vi "PathDrawerMain.vi"() -> ()   [LabVIEW 2017]
uses:
  Shared/PathFileData.ctl
  Shared/RobotNeededPathData.ctl
panel:
  in  "Tab Control":enum32{"Path", "Load/Save"}(tab)
  in  "Points":cluster{dbl, dbl}[](array[cluster])=[{46.0, 206.0}, {72.0, 199.0}, {97.0, 267.0}, {149.0, 262.0}]
  in  "Roundedness":dbl(slide)=0.7875252525252525 scale=0.6..0.995
  in  "RobotLength":dbl=40.0
  in  "RobotWidth":dbl=30.0
  in  "CenterOfRotYOffset":dbl=20.0
  in  "PointSpacing":dbl=12.0 min=1.0 format="%#_13g"
  in  "Starting Position Preset":enum16{"1", "2", "3", "4", "No Preset"}(ring)=enum."3"
  in  "Flip Path":bool
  in  "MaxVel":dbl=100.0 format="%#_13g"
  in  "MaxAccel":dbl=100.0 format="%#_13g"
  in  "LocalTempPaths":i32(listbox)
  out "standard output":string
  in  "ExportToLocal":bool
  in  "LoadFromLocal":bool
  in  "ExportToRobot":bool
  in  "LoadAllFromRobot":bool
  in  "LocalPaths":i32(listbox)
  out "standard error":string
  in  "LocalFileNames":string[](array[string])
  in  "Stop":bool
  out "Path Drawer":T1(plugin-control)
  # "MORE INSTRUCTIONS"
  # "Use a preset if your path starts\nat one of the presets. \n\n(Click it multiple times please)"
  # "Includes bumpers"
  # "Relative to outside face of\nback bumber of robot"
  # "INSTRUCTIONS"
  # "The red line is the path that the robot recieves. Everything else is to help create that path\n\nUse the multi-line tool to draw a path. Double click to stop drawing.\nHover over a node and press backspace to remove it.\nPress I to insert a new node (at the end of the path only, for now)\n\nUse the contols to input robot width, height, and center of rotation offset,\nHow far apart the points in the \"real world units\" path are,\nWhether the robot travels on the left or right of your green lines, and\nthe roundedness of the path. (Note: point spacing affects roundedness)\n\nYou can manually edit the green node's location in the path with the Points array,\nor drag the nodes on the image\n\nPress Export To File and enter the file name (no extension) to save the path to a file in the\nThisVIsDirectory\\Paths\\ folder\n\nIf you acidentally clear your path press Z quickly to get it back"
  # "Responses of CMDs run"
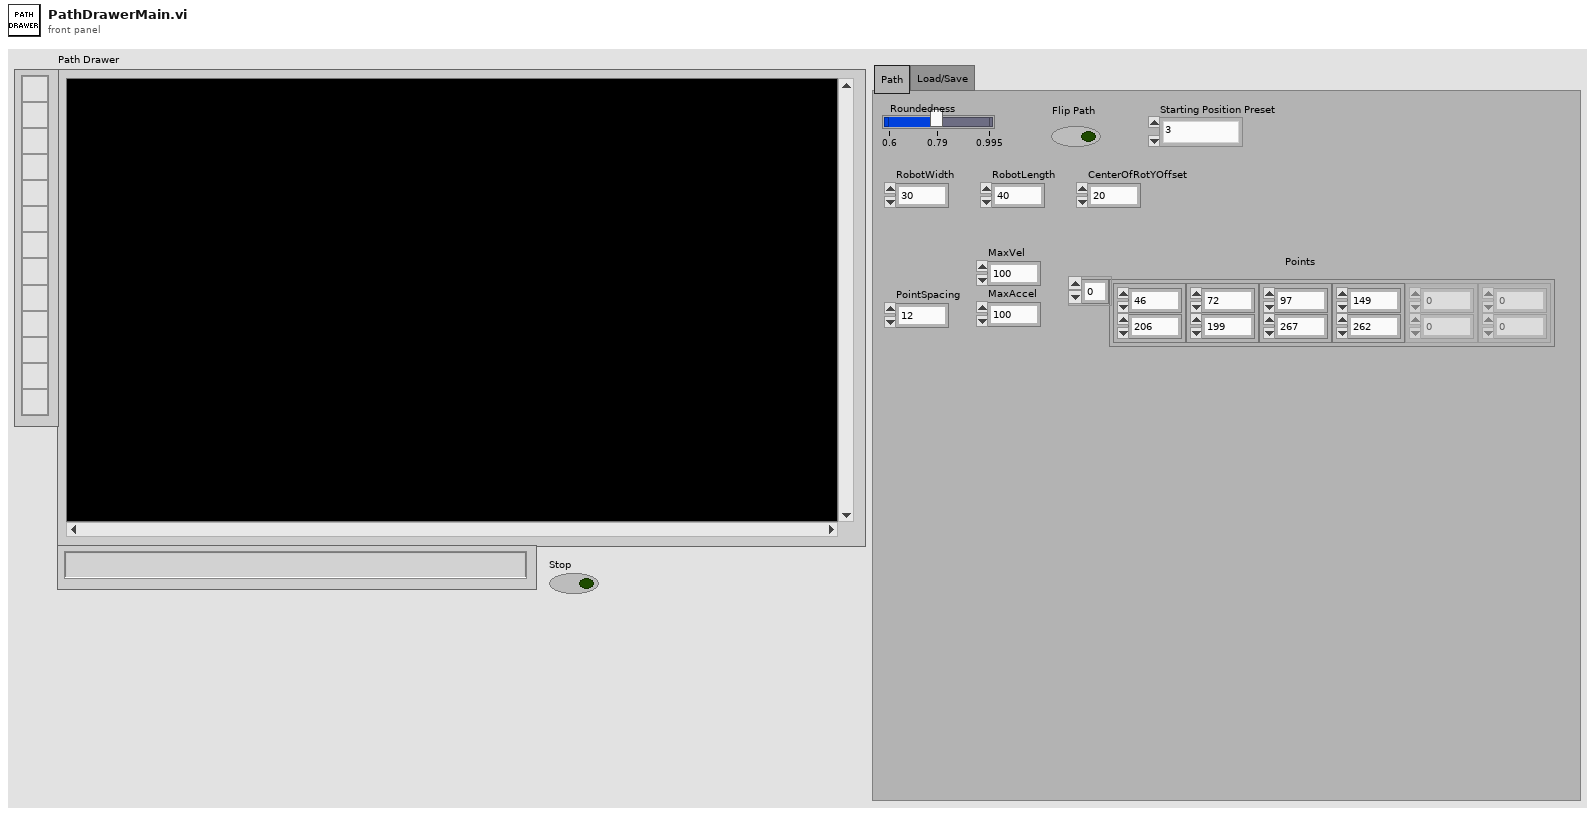
[diagram p1: front panel]
types:
  T1 = typedef "IMAQ Image.ctl" = refnum<image>
  T2 = typedef "Image Type" = u32
  T3 = typedef "PathFileData.ctl" = cluster{"RobotNeeded":T4, "Meta":cluster{"Path (px)":cluster{i32, i32}[], "RobotWidth":dbl, "RobotLength":dbl, "CenterOfRotYOffset":dbl, "Roundedness":dbl, "StartingPositionPreset":u32, "PathName":string}}
  T4 = typedef "RobotNeededPathData.ctl" = cluster{"Path":cluster{dbl, dbl}[], "MaxVel":dbl, "MaxAccel":dbl, "Backwards?":bool, "PointSpacing":dbl}
  T5 = cluster{"Global Rectangle":i32[], "Contours":cluster{"Contour Type":u32, "ROI Type":u32, "Points":i32[]}[]}
  T6 = cluster{"Contour Type":u32, "ROI Type":u32, "Points":i32[]}[]
  T7 = cluster{"Path (px)":cluster{i32, i32}[], "RobotWidth":dbl, "RobotLength":dbl, "CenterOfRotYOffset":dbl, "Roundedness":dbl, "StartingPositionPreset":u32, "PathName":string}
  T8 = cluster{"Contour Type":u32, "ROI Type":u32, "Points":i32[]}
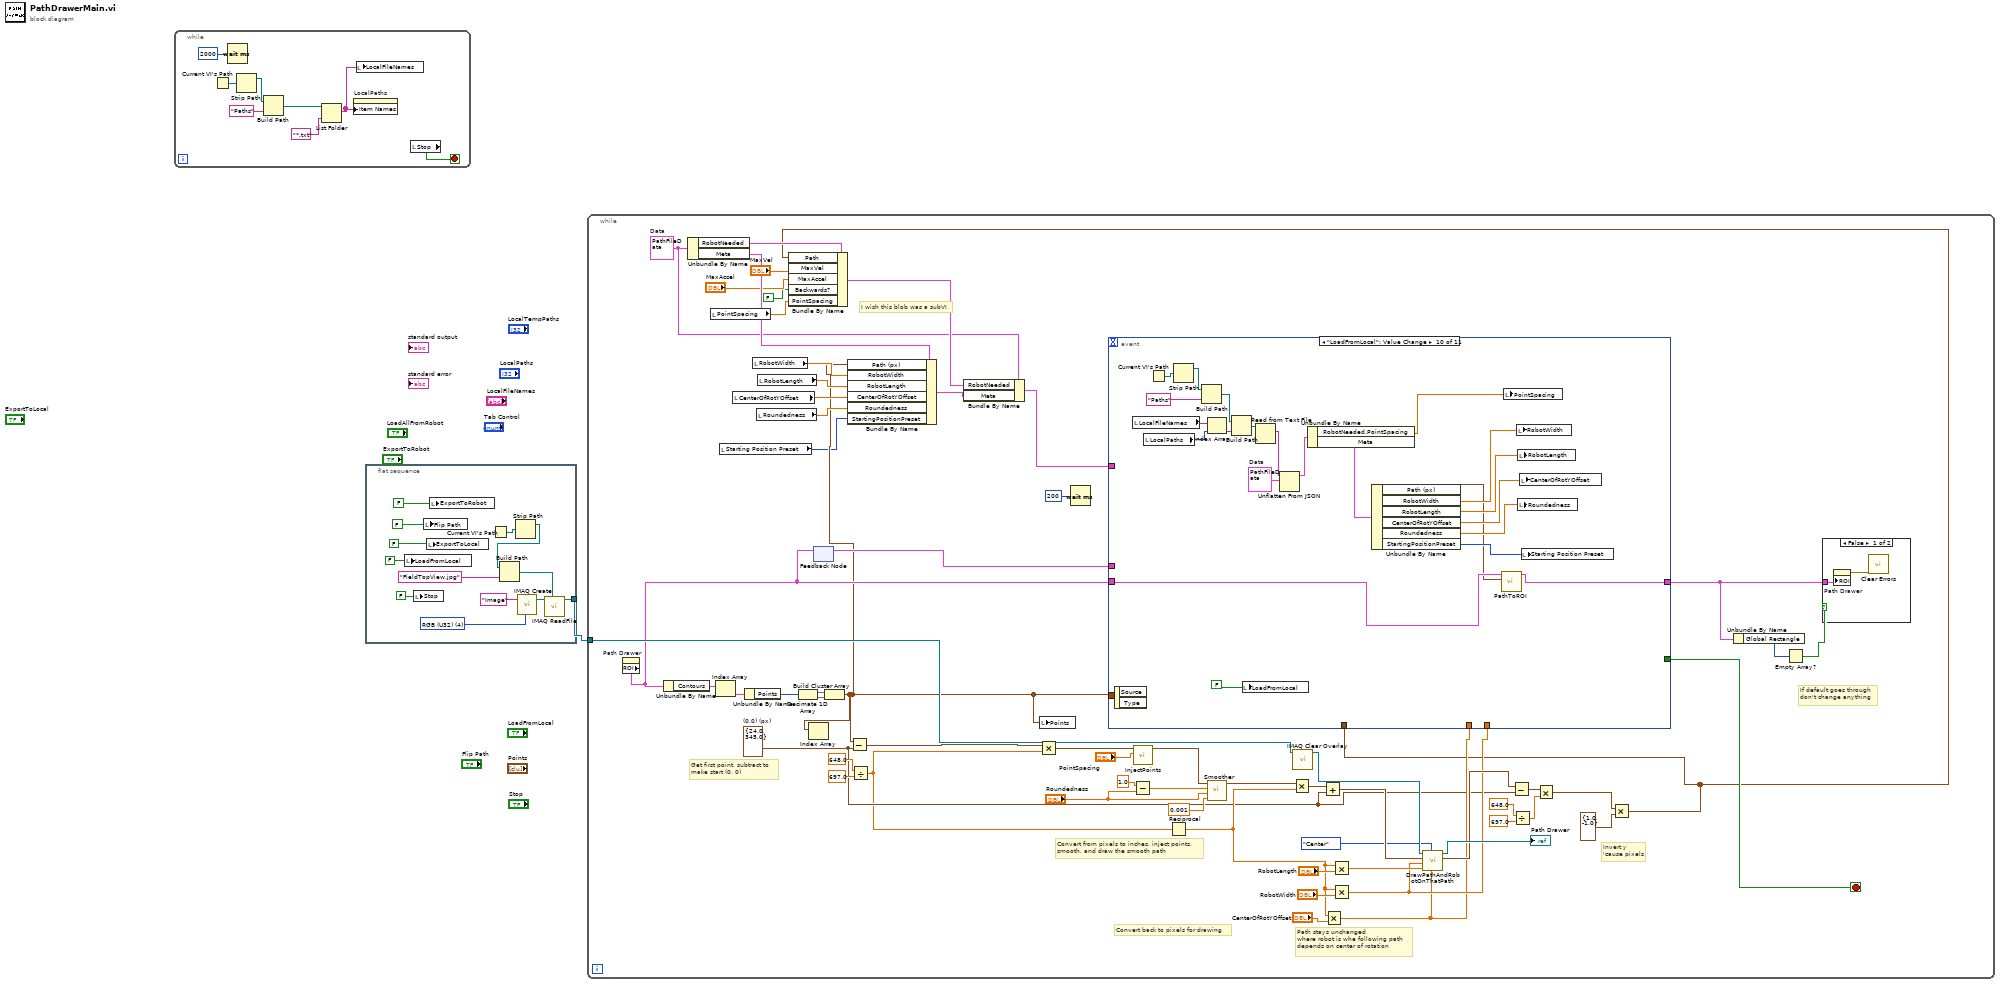
[diagram p0: block diagram]
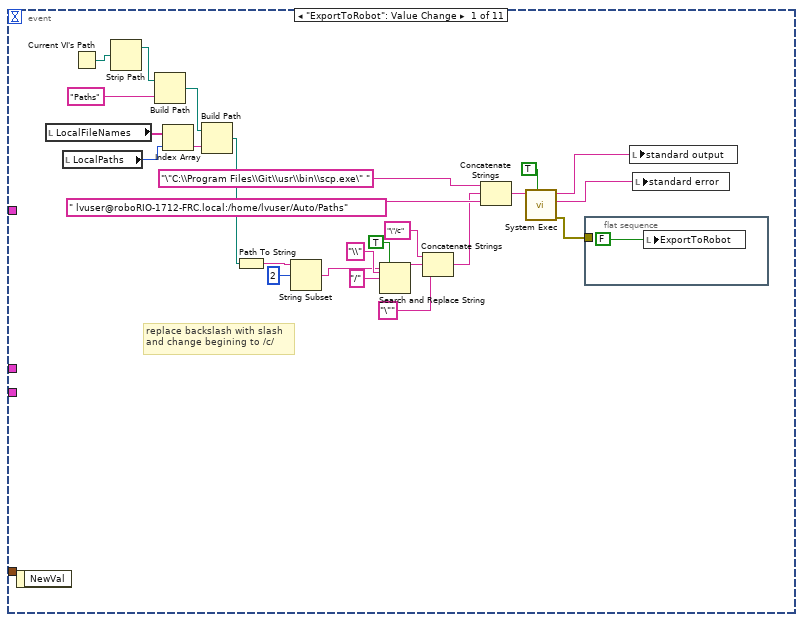
[diagram p3: hidden frame]
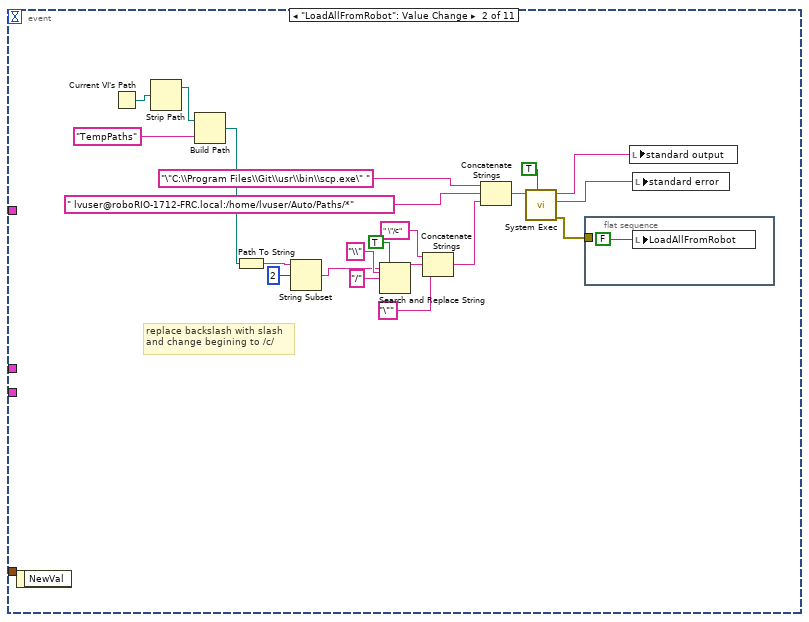
[diagram p4: hidden frame]
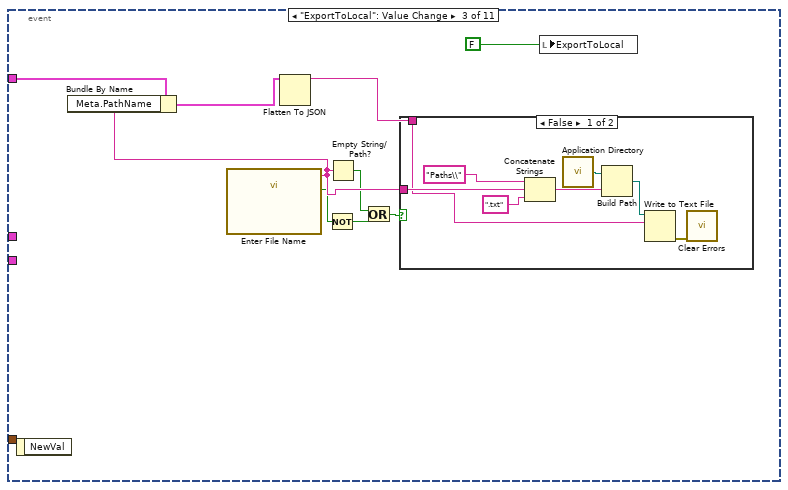
[diagram p5: hidden frame]
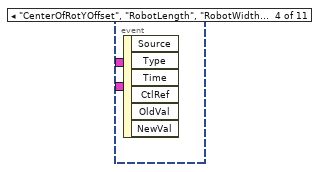
[diagram p7: hidden frame]
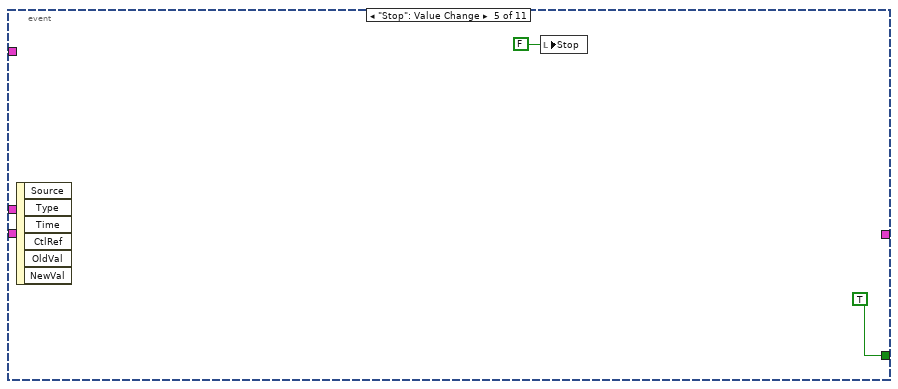
[diagram p8: hidden frame]
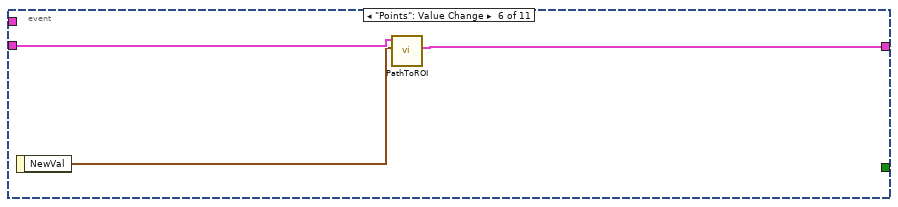
[diagram p9: hidden frame]
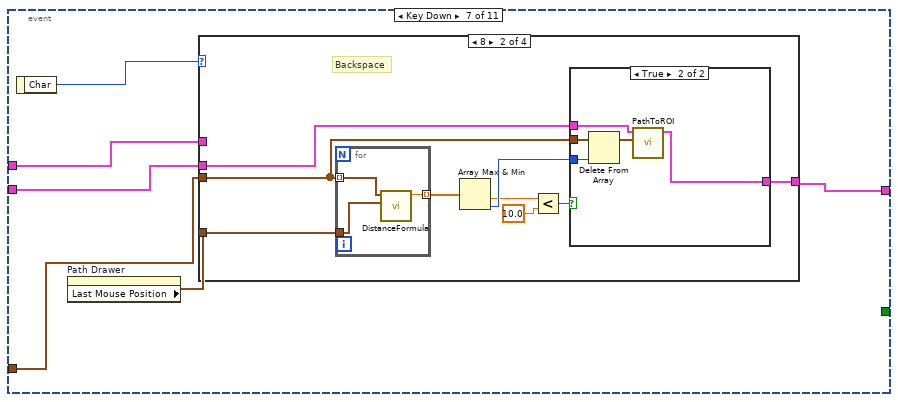
[diagram p10: hidden frame]
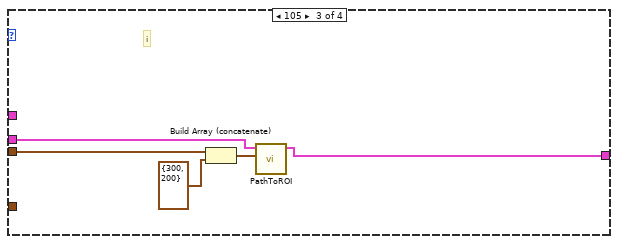
[diagram p13: hidden frame]
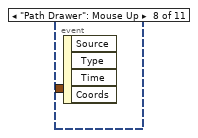
[diagram p15: hidden frame]
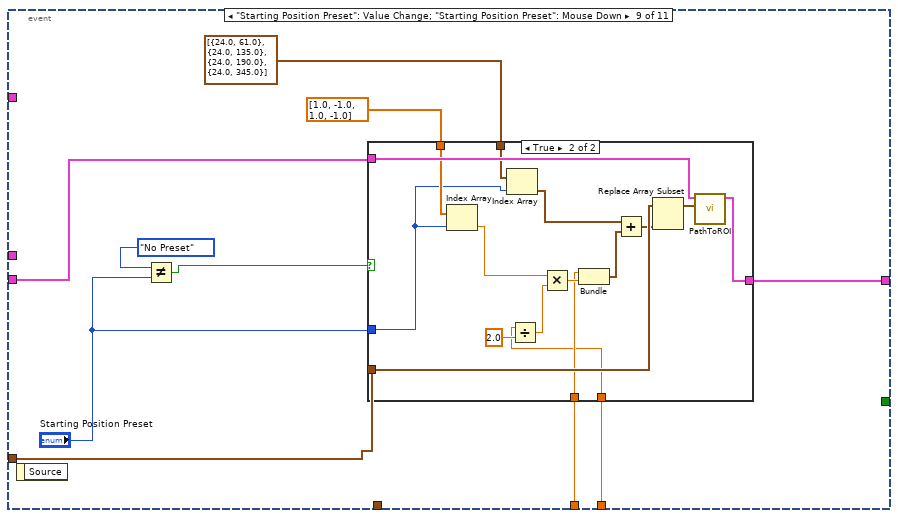
[diagram p16: hidden frame]
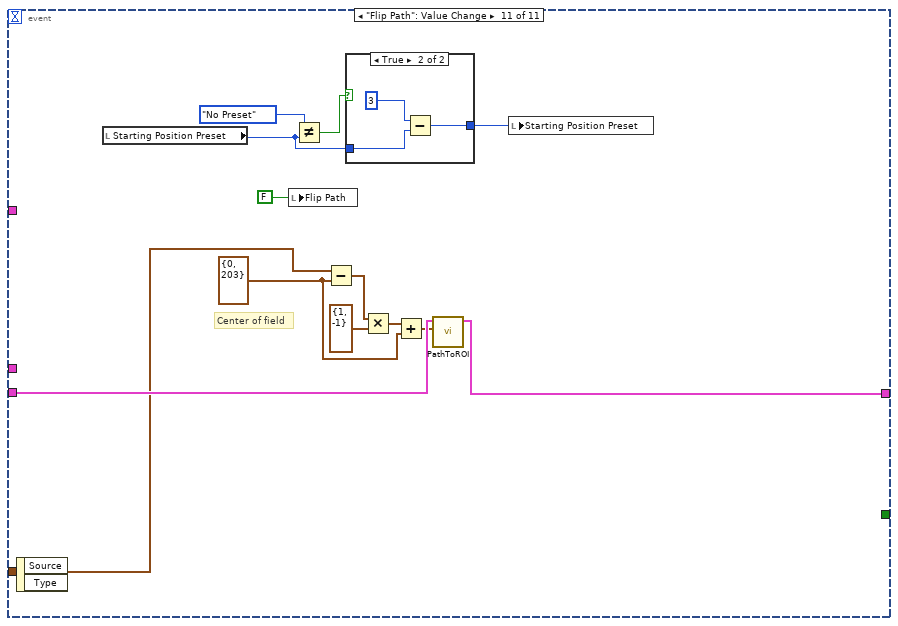
[diagram p18: hidden frame]
diagram:
  n1 = while {
    stop <- w8 stop-if-true
    n2 = Current VI's Path() -> (path=w3:path)
    n3 = Wait (ms)(milliseconds to wait=u32 2000) -> ()  [unwired: 1 out]
    n4 = Strip Path(path=w3) -> (stripped path=w2:path)  [unwired: 1 out]
    n5 = Build Path(base path=w2, name or relative path="Paths") -> (appended path=w5:path)
    n6 = List Folder(path=w5, pattern="*.txt") -> (filenames=w7:string[])  [unwired: 2 in, 3 out]
    n7 = property on="LocalPaths" class="LstBox (strict)"("Item Names"=w7) -> ()  [unwired: 2 in, 2 out]
    n8 = local write "LocalFileNames"(w7) -> ()
    n9 = local read "Stop"() -> (w8:bool)
  }
  n10 = flat-sequence {
    tunnel: [w17] -> w1
    frame #0 {
      w19 = T2 4 items=["Grayscale (U8)", "Grayscale (I16)", "Grayscale (SGL)", "Complex (CSG)", "RGB (U32)", "HSL (U32)", "RGB (U64)", "Grayscale (U16)"] ("Image Type")
      n11 = local write "LoadFromLocal"(FALSE ("Export To File")) -> ()
      n12 = local write "Stop"(FALSE ("Stop")) -> ()
      n13 = local write "Flip Path"(FALSE ("Export To File")) -> ()
      n14 = local write "ExportToLocal"(FALSE ("Export To File")) -> ()
      n15 = local write "ExportToRobot"(FALSE ("Export To File")) -> ()
      n16 = Current VI's Path() -> (path=w11:path)
      n17 = Strip Path(path=w11) -> (stripped path=w10:path)  [unwired: 1 out]
      n18 = Build Path(base path=w10, name or relative path="FieldTopView.jpg") -> (appended path=w21:path)
      n19 = call "IMAQ Create"("Image Name"="Image", "Image Type"=w19) -> ("New Image"=w18:T1)  [unwired: 3 in, 1 out]
      n20 = call "IMAQ ReadFile"("File Path"=w21, "Image"=w18) -> ("Image Out"=w17:T1)  [unwired: 5 in, 4 out]
    }
  }
  n21 = while {
    tunnel: w1 -> [w78]
    stop <- w47 stop-if-true
    w28 = cluster{dbl, dbl} {24.0, 345.0}  # (0,0) (px)
    w34 = T3 {"RobotNeeded"={"Path"=[], "MaxVel"=0.0, "MaxAccel"=0.0, "Backwards?"=FALSE, "PointSpacing"=0.0}, "Meta"={"Path (px)"=[], "RobotWidth"=0.0, "RobotLength"=0.0, "CenterOfRotYOffset"=0.0, "Roundedness"=0.0, "StartingPositionPreset"=2, "PathName"=""}}  # Data
    # "Invert y\n'cause pixels"
    # "I wish this blob was a subVI"
    # "Path stays unchanged\nwhere robot is whe following path\ndepends on center of rotation"
    # "Convert back to pixels for drawing"
    # "If default goes through\ndon't change anything"
    # "Convert from pixels to inches, inject points,\nsmooth, and draw the smooth path"
    # "Get first point, subtract to\nmake start (0, 0)"
    n22 = property on="Path Drawer" class="ImageControl"() -> ("ROI"=w57:T5)  [unwired: 2 in, 2 out]
    n23 = Unbundle By Name(w57) -> ("Contours"=w84:T6)
    n24 = Unbundle By Name(w34) -> ("RobotNeeded"=w39:T4, "Meta"=w40:T7)
    n25 = local read "PointSpacing"() -> (w23:dbl)
    n26 = Index Array(array=w84) -> (element=w79:T8)  [unwired: 1 in]
    n27 = local read "Starting Position Preset"() -> (w24:enum16{"1", "2", "3", "4", "No Preset"})
    n28 = local read "CenterOfRotYOffset"() -> (w44:dbl)
    n29 = Unbundle By Name(w79) -> ("Points"=w73:i32[])
    n30 = local read "RobotWidth"() -> (w42:dbl)
    n31 = local read "Roundedness"() -> (w45:dbl)
    n32 = local read "RobotLength"() -> (w43:dbl)
    n33 = Decimate 1D Array(w73) -> (w83:i32[], w82:i32[])
    n34 = feedback-in #1(w57) -> ()
    n35 = feedback #1() -> (w56:T5)  [unwired: 1 in]
    n36 = Build Cluster Array(w83, w82) -> (w26:cluster{i32, i32}[])
    n37 = Index Array(array=w26) -> ()  [unwired: 1 in, 1 out]
    n38 = Bundle By Name(cluster=w40, "Path (px)"=w26, "RobotWidth"=w42, "RobotLength"=w43, "CenterOfRotYOffset"=w44, "Roundedness"=w45, "StartingPositionPreset"=w24) -> (w41:T7)
    n39 = Subtract(x=w26, y=w28) -> (x-y=w74:cluster{dbl, dbl}[])
    n40 = Divide(x=648.0, y=697.0) -> (x/y=w25:dbl)
    n41 = Multiply(x=w74, y=w25) -> (x*y=w58:cluster{dbl, dbl}[])
    n42 = local write "Points"(w26) -> ()
    n43 = Wait (ms)(milliseconds to wait=u32 200) -> ()  [unwired: 1 out]
    n44 = call "InjectPoints.vi"("Distance"="PointSpacing", "Path"=w58) -> ("Path out"=w76:cluster{dbl, dbl}[])  [unwired: 9 in]
    n45 = Subtract(x=1.0, y="Roundedness") -> (x-y=w71:dbl)
    n46 = Reciprocal(x=w25) -> (1/x=w54:dbl)
    n47 = call "Smoother.vi"("tolerance"=0.001, "B"="Roundedness", "A"=w71, "Path"=w76) -> ("SmoothPath"=w66:cluster{dbl, dbl}[])  [unwired: 7 in]
    n48 = Multiply(x=w66, y=w54) -> (x*y=w75:cluster{dbl, dbl}[])
    n49 = call "IMAQ Clear Overlay"("Image"=w78) -> ("Image Out"=w51:T1)  [unwired: 9 in, 1 out]
    n50 = Add(x=w75, y=w28) -> (x+y=w50:cluster{dbl, dbl}[])
    n51 = Multiply(x=w54, y="CenterOfRotYOffset") -> (x*y=w31:dbl)
    n52 = Multiply(x=w54, y="RobotLength") -> (x*y=w49:dbl)
    n53 = Multiply(x=w54, y="RobotWidth") -> (x*y=w32:dbl)
    n54 = call "DrawPathAndRobotOnThatPath.vi"("CenterOfRotYOffset (px)"=w31, "PathMode"=enum16{"Left", "Right", "Center"}."Center", "RobotLength (px)"=w49, "RobotWidth (px)"=w32, "Path (px)"=w50, "Image In"=w51) -> ("NewPath (px)"=w52:cluster{dbl, dbl}[], "Image Out"=→"Path Drawer":T1)  [unwired: 4 in]
    n55 = Subtract(x=w52, y=w28) -> (x-y=w59:cluster{dbl, dbl}[])
    n56 = Divide(x=648.0, y=697.0) -> (x/y=w60:dbl)
    n57 = Multiply(x=w59, y=w60) -> (x*y=w30:cluster{dbl, dbl}[])
    n58 = Multiply(x=w30, y=cluster{dbl, dbl} {1.0, -1.0}) -> (x*y=w27:cluster{dbl, dbl}[])
    n59 = Bundle By Name(cluster=w39, "Path"=w27, "MaxVel"="MaxVel", "MaxAccel"="MaxAccel", "Backwards?"=FALSE, "PointSpacing"=w23) -> (w38:T4)
    n60 = Bundle By Name(cluster=w34, "RobotNeeded"=w38, "Meta"=w41) -> (w33:T3)
    n61 = event shown="[9] \"LoadFromLocal\": Value Change" {
      selector: _ -> [_ _ _ _ _ _ _ _ _ _ _]
      dyn-events: _ -> [_ _ _ _ _ _ _ _ _ _ _]
      timeout: _ -> [_ _ _ _ _ _ _ _ _ _ _]
      tunnel: w57 -> [_ _ _ _ _ w156 w162 _ w196 w220 w247]
      tunnel: [_ _ _ _ _ w155 w159 _ w197 w234 w246] -> w46
      tunnel: w27 -> [_ _ _ _ _ _ _ _ _ _ _]
      tunnel: w56 -> [_ _ _ _ _ _ w158 _ _ _ _]
      tunnel: w26 -> [_ _ _ _ _ _ w157 _ w190 _ w241]
      tunnel: w31 -> [_ _ _ _ _ _ _ _ w192 _ _]
      tunnel: w32 -> [_ _ _ _ _ _ _ _ w191 _ _]
      tunnel: [_ _ _ _ TRUE ("Stop") _ _ _ _ _ _] -> w47
      tunnel: w33 -> [_ _ w141 _ _ _ _ _ _ _ _]
      event "ExportToRobot": Value Change {
        # "replace backslash with slash\nand change begining to /c/"
        n62 = event-data() -> ()  [unwired: 1 in, 1 out]
        n63 = local read "LocalFileNames"() -> (w93:string[])
        n64 = local read "LocalPaths"() -> (w94:i32)
        n65 = Current VI's Path() -> (path=w96:path)
        n66 = Strip Path(path=w96) -> (stripped path=w95:path)  [unwired: 1 out]
        n67 = Build Path(base path=w95, name or relative path="Paths") -> (appended path=w98:path)
        n68 = Index Array(array=w93, index=w94) -> (element=w97:string)
        n69 = Build Path(base path=w98, name or relative path=w97) -> (appended path=w91:path)
        n70 = Path To String(path=w91) -> (string=w104:string)
        n71 = String Subset(string=w104, offset (0)=2) -> (substring=w102:string)  [unwired: 1 in]
        n72 = Search and Replace String(replace all?=TRUE ("replace all? (F)"), input string=w102, search string="\\", replace string="/" ("replace string (\"\")")) -> (result string=w101:string)  [unwired: 4 in, 3 out]
        n73 = Concatenate Strings("\"/c" ("string"), w101, "\"" ("string")) -> (w99:string)
        n74 = Concatenate Strings("\"C:\\Program Files\\Git\\usr\\bin\\scp.exe\" " ("command line"), w99, " lvuser@roboRIO-1712-FRC.local:/home/lvuser/Auto/Paths" ("string")) -> (w108:string)
        n75 = call <vilib>:"System Exec.vi"("wait until completion? (T)"=TRUE, "command line"=w108) -> ("error out"=w89:errorcluster, "standard error"=w87:string, "standard output"=w88:string)  [unwired: 6 in, 1 out]
        n76 = flat-sequence {
          tunnel: w89 -> [_]
          frame #0 {
            n77 = local write "ExportToRobot"(FALSE ("Export To File")) -> ()
          }
        }
        n78 = local write "standard output"(w88) -> ()
        n79 = local write "standard error"(w87) -> ()
      }
      event "LoadAllFromRobot": Value Change {
        # "replace backslash with slash\nand change begining to /c/"
        n80 = event-data() -> ()  [unwired: 1 in, 1 out]
        n81 = Current VI's Path() -> (path=w122:path)
        n82 = Strip Path(path=w122) -> (stripped path=w121:path)  [unwired: 1 out]
        n83 = Build Path(base path=w121, name or relative path="TempPaths") -> (appended path=w115:path)
        n84 = Path To String(path=w115) -> (string=w127:string)
        n85 = String Subset(string=w127, offset (0)=2) -> (substring=w125:string)  [unwired: 1 in]
        n86 = Search and Replace String(replace all?=TRUE ("replace all? (F)"), input string=w125, search string="\\", replace string="/" ("replace string (\"\")")) -> (result string=w124:string)  [unwired: 4 in, 3 out]
        n87 = Concatenate Strings(" \"/c" ("string"), w124, "\"" ("string")) -> (w113:string)
        n88 = Concatenate Strings("\"C:\\Program Files\\Git\\usr\\bin\\scp.exe\" " ("command line"), " lvuser@roboRIO-1712-FRC.local:/home/lvuser/Auto/Paths/*" ("string"), w113) -> (w131:string)
        n89 = call <vilib>:"System Exec.vi"("wait until completion? (T)"=TRUE, "command line"=w131) -> ("error out"=w118:errorcluster, "standard error"=w116:string, "standard output"=w117:string)  [unwired: 6 in, 1 out]
        n90 = flat-sequence {
          tunnel: w118 -> [_]
          frame #0 {
            n91 = local write "LoadAllFromRobot"(FALSE ("Export To File")) -> ()
          }
        }
        n92 = local write "standard output"(w117) -> ()
        n93 = local write "standard error"(w116) -> ()
      }
      event "ExportToLocal": Value Change {
        n94 = event-data() -> ()  [unwired: 1 in, 1 out]
        n95 = call "Enter File Name"() -> ("File Name"=w140:string, "Enter"=w136:bool)  [unwired: 17 in, 1 out]
        n96 = Bundle By Name(cluster=w141, "Meta.PathName"=w140) -> (w139:T3)
        n97 = Flatten To JSON(anything=w139) -> (JSON string=w142:string)  [unwired: 2 in, 1 out]
        n98 = Not(x=w136) -> (.not. x?=w135:bool)
        n99 = Empty String/Path?(string/path=w140) -> (empty?=w138:bool)
        n100 = Or(x=w138, y=w135) -> (x .or. y?=w137:bool)
        n101 = case shown="False" w137 {
          tunnel: w140 -> [w145 _]
          tunnel: w142 -> [w144 _]
          frame False {
            n102 = Concatenate Strings("Paths\\" ("name or relative path"), w145, ".txt" ("string")) -> (w151:string)
            n103 = call <vilib>:"Application Directory.vi"() -> ("Application Directory"=w150:path)
            n104 = Build Path(base path=w150, name or relative path=w151) -> (appended path=w147:path)
            n105 = Write to Text File(file (use dialog)=w147, text=w144) -> (error out=w148:errorcluster)  [unwired: 2 in, 2 out]
            n106 = call <vilib>:"Clear Errors.vi"("error in (no error)"=w148) -> ()  [unwired: 5 in, 2 out]
          }
          frame True {
          }
        }
        n107 = local write "ExportToLocal"(FALSE ("Export To File")) -> ()
      }
      event "CenterOfRotYOffset", "RobotLength", "RobotWidth", "PointSpacing", "Roundedness": Value Change {
        n108 = event-data() -> ()  [unwired: 1 in, 6 out]
      }
      event "Stop": Value Change {
        n109 = event-data() -> ()  [unwired: 1 in, 6 out]
        n110 = local write "Stop"(FALSE ("Stop")) -> ()
      }
      event "Points": Value Change {
        n111 = event-data() -> ("NewVal"=w154:cluster{dbl, dbl}[])  [unwired: 1 in]
        n112 = call "PathToROI.vi"("Path In"=w154, "ROI In"=w156) -> ("ROI Out"=w155:T5)  [unwired: 9 in]
      }
      event Key Down {
        n113 = event-data() -> ("Char"=w161:i16)  [unwired: 1 in]
        n114 = property on="Path Drawer" class="ImageControl"() -> ("Last Mouse Position"=w160:cluster{"X":i32, "Y":i32})  [unwired: 2 in, 2 out]
        n115 = case shown="8" w161 {
          tunnel: w162 -> [w163 w172 w184 _]
          tunnel: w157 -> [_ w171 w186 _]
          tunnel: w160 -> [_ w165 _ _]
          tunnel: [w163 w164 w182 w187] -> w159
          tunnel: w158 -> [_ _ _ w187]
          frame 0, Default {
          }
          frame 8 {
            # "Backspace"
            n116 = for {
              tunnel: w171 -> [w181] mode=indexing
              tunnel: [w180] -> w170 mode=indexing
              tunnel: w165 -> [w179]
              n117 = call "DistanceFormula.vi"("Point 2"=w179, "Point 1"=w181) -> ("Distance"=w180:dbl)  [unwired: 9 in]
            }
            n118 = Array Max & Min(array=w170) -> (min value=w168:dbl, min index (indices)=w169:i32)  [unwired: 2 out]
            n119 = Less?(x=w168, y=10.0) -> (x < y?=w166:bool)
            n120 = case shown="True" w166 {
              tunnel: w169 -> [_ w178]
              tunnel: w171 -> [_ w177]
              tunnel: w172 -> [w173 w175]
              tunnel: [w173 w174] -> w164
              frame False {
              }
              frame True {
                n121 = Delete From Array(array=w177, index=w178) -> (array with subset deleted=w176:cluster{i32, i32}[])  [unwired: 1 in, 1 out]
                n122 = call "PathToROI.vi"("Path In"=w176, "ROI In"=w175) -> ("ROI Out"=w174:T5)  [unwired: 9 in]
              }
            }
          }
          frame 105 {
            # "i"
            n123 = Build Array (concatenate)(w186, cluster{i32, i32} {300, 200}) -> (w185:cluster{i32, i32}[])
            n124 = call "PathToROI.vi"("Path In"=w185, "ROI In"=w184) -> ("ROI Out"=w182:T5)  [unwired: 9 in]
          }
          frame 122 {
            # "Restore last ROI"
            # "Z"
          }
        }
      }
      event "Path Drawer": Mouse Up {
        n125 = event-data() -> ()  [unwired: 1 in, 4 out]
      }
      event "Starting Position Preset": Value Change; "Starting Position Preset": Mouse Down {
        n126 = event-data() -> ()  [unwired: 1 in, 1 out]
        n127 = Not Equal?(x=enum16{"1", "2", "3", "4", "No Preset"}."No Preset" ("y"), y="Starting Position Preset") -> (x != y?=w194:bool)
        n128 = case shown="True" w194 {
          tunnel: [_ w213] -> w197
          tunnel: w196 -> [_ w212]
          tunnel: w190 -> [_ w210]
          tunnel: "Starting Position Preset" -> [_ w199]
          tunnel: w192 -> [_ w204]
          tunnel: w191 -> [_ w203]
          tunnel: cluster{dbl, dbl}[] [{24.0, 61.0}, {24.0, 135.0}, {24.0, 190.0}, {24.0, 345.0}] -> [_ w202]
          tunnel: dbl[] [1.0, -1.0, 1.0, -1.0] -> [_ w200]
          frame False {
          }
          frame True {
            n129 = Index Array(array=w200, index=w199) -> (element=w198:dbl)
            n130 = Index Array(array=w202, index=w199) -> (element=w201:cluster{dbl, dbl})
            n131 = Divide(x=w203, y=2.0) -> (x/y=w207:dbl)
            n132 = Multiply(x=w198, y=w207) -> (x*y=w206:dbl)
            n133 = Bundle(w204, w206) -> (w205:cluster{dbl, dbl})  [unwired: 1 in]
            n134 = Add(x=w201, y=w205) -> (x+y=w209:cluster{dbl, dbl})
            n135 = Replace Array Subset(array=w210, new element=w209) -> (w211:cluster{i32, i32}[])  [unwired: 1 in]
            n136 = call "PathToROI.vi"("Path In"=w211, "ROI In"=w212) -> ("ROI Out"=w213:T5)  [unwired: 9 in]
          }
        }
      }
      event "LoadFromLocal": Value Change {
        w231 = T3 {"RobotNeeded"={"Path"=[], "MaxVel"=0.0, "MaxAccel"=0.0, "Backwards?"=FALSE, "PointSpacing"=0.0}, "Meta"={"Path (px)"=[], "RobotWidth"=0.0, "RobotLength"=0.0, "CenterOfRotYOffset"=0.0, "Roundedness"=0.0, "StartingPositionPreset"=2, "PathName"=""}}  # Data
        n137 = event-data() -> ()  [unwired: 1 in, 2 out]
        n138 = local read "LocalFileNames"() -> (w215:string[])
        n139 = local read "LocalPaths"() -> (w216:i32)
        n140 = Current VI's Path() -> (path=w218:path)
        n141 = Strip Path(path=w218) -> (stripped path=w217:path)  [unwired: 1 out]
        n142 = Build Path(base path=w217, name or relative path="Paths") -> (appended path=w223:path)
        n143 = Index Array(array=w215, index=w216) -> (element=w222:string)
        n144 = Build Path(base path=w223, name or relative path=w222) -> (appended path=w221:path)
        n145 = local write "LoadFromLocal"(FALSE ("Export To File")) -> ()
        n146 = Read from Text File(file (use dialog)=w221) -> (text=w233:string)  [unwired: 3 in, 3 out]
        n147 = Unflatten From JSON(JSON string=w233, type and defaults=w231) -> (value=w230:T3)  [unwired: 5 in, 1 out]
        n148 = Unbundle By Name(w230) -> ("RobotNeeded.PointSpacing"=w214:dbl, "Meta"=w229:T7)
        n149 = Unbundle By Name(w229) -> ("Path (px)"=w219:cluster{i32, i32}[], "RobotWidth"=w224:dbl, "RobotLength"=w225:dbl, "CenterOfRotYOffset"=w228:dbl, "Roundedness"=w227:dbl, "StartingPositionPreset"=w226:u32)
        n150 = call "PathToROI.vi"("Path In"=w219, "ROI In"=w220) -> ("ROI Out"=w234:T5)  [unwired: 9 in]
        n151 = local write "PointSpacing"(w214) -> ()
        n152 = local write "RobotWidth"(w224) -> ()
        n153 = local write "RobotLength"(w225) -> ()
        n154 = local write "Roundedness"(w227) -> ()
        n155 = local write "CenterOfRotYOffset"(w228) -> ()
        n156 = local write "Starting Position Preset"(w226) -> ()
      }
      event "Flip Path": Value Change {
        w243 = cluster{i32, i32} {0, 203}
        # "Center of field"
        n157 = event-data() -> ()  [unwired: 1 in, 2 out]
        n158 = local read "Starting Position Preset"() -> (w237:enum16{"1", "2", "3", "4", "No Preset"})
        n159 = local write "Flip Path"(FALSE ("Export To File")) -> ()
        n160 = Not Equal?(x=enum16{"1", "2", "3", "4", "No Preset"}."No Preset", y=w237) -> (x != y?=w238:bool)
        n161 = Subtract(x=w241, y=w243) -> (x-y=w242:cluster{i32, i32}[])
        n162 = case shown="True" w238 {
          tunnel: w237 -> [w249 w252]
          tunnel: [w249 w250] -> w236
          frame False {
          }
          frame True {
            n163 = Subtract(x=3, y=w252) -> (x-y=w250:i32)
          }
        }
        n164 = Multiply(x=w242, y=cluster{i32, i32} {1, -1}) -> (x*y=w244:cluster{i32, i32}[])
        n165 = Add(x=w244, y=w243) -> (x+y=w240:cluster{i32, i32}[])
        n166 = call "PathToROI.vi"("Path In"=w240, "ROI In"=w247) -> ("ROI Out"=w246:T5)  [unwired: 9 in]
        n167 = local write "Starting Position Preset"(w236) -> ()
      }
    }
    n168 = Unbundle By Name(w46) -> ("Global Rectangle"=w68:i32[])
    n169 = Empty Array?(array=w68) -> (empty?=w67:bool)
    n170 = case shown="False" w67 {
      tunnel: w46 -> [w85 _]
      frame False {
        n171 = property on="Path Drawer" class="ImageControl"("ROI"=w85) -> (error out=w86:errorcluster)  [unwired: 2 in, 1 out]
        n172 = call <vilib>:"Clear Errors.vi"("error in (no error)"=w86) -> ()  [unwired: 5 in, 2 out]
      }
      frame True {
      }
    }
  }
